vi "GetSubarrayOfCircularBuffer.vi"(8 "initialized array":waveform(dbl)[](array[waveform]), 9 "buffer size":i32, 10 "subset size":i32, 11 "start index":i32) -> (2 "initialized array 2":waveform(dbl)[](array[waveform]))   [LabVIEW 2016]
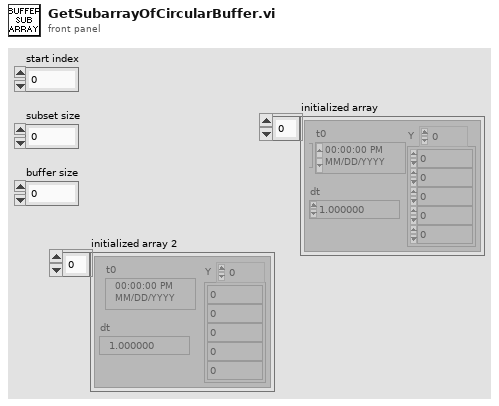
[diagram p1: front panel]
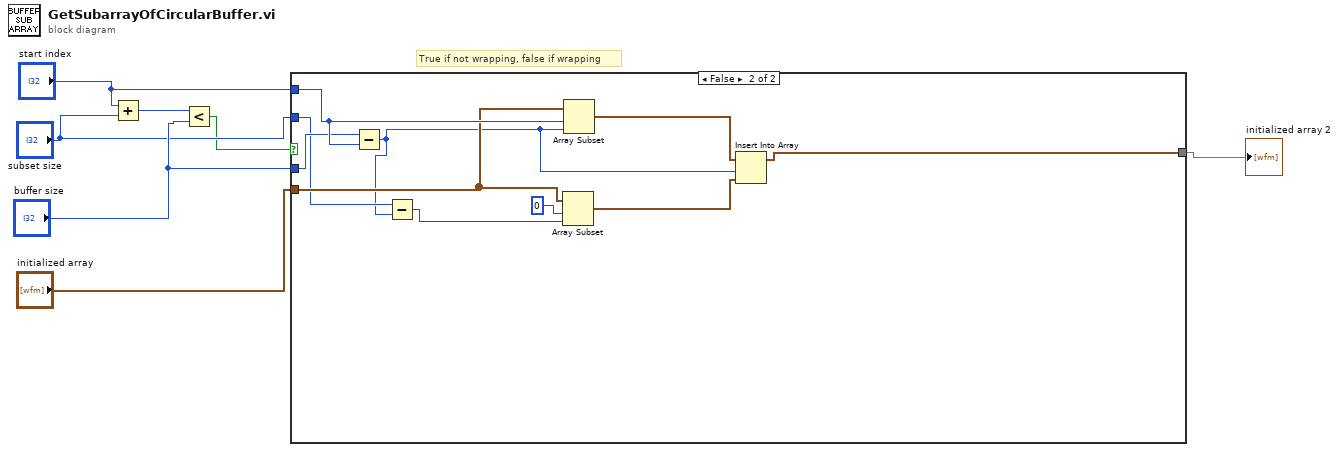
[diagram p0: block diagram]
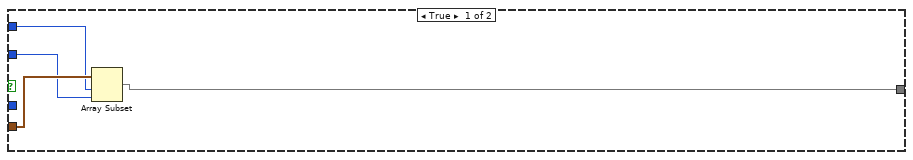
[diagram p2: hidden frame]
diagram:
  # "True if not wrapping, false if wrapping"
  n1 = Add(x="start index", y="subset size") -> (x+y=w3:i32)
  n2 = Less?(x=w3, y="buffer size") -> (x < y?=w4:bool)
  n3 = case shown="False" w4 {
    tunnel: "initialized array" -> [w11 w19]
    tunnel: "start index" -> [w10 w21]
    tunnel: "subset size" -> [w9 w17]
    tunnel: "buffer size" -> [_ w20]
    tunnel: [w8 w12] -> w1
    frame True {
      n4 = Array Subset(array=w11, index=w10, length=w9) -> (w8:waveform(dbl)[])
    }
    frame False, Default {
      n5 = Subtract(x=w20, y=w21) -> (x-y=w14:i32)
      n6 = Subtract(x=w17, y=w14) -> (x-y=w16:i32)
      n7 = Array Subset(array=w19, index=0, length=w16) -> (w13:waveform(dbl)[])
      n8 = Array Subset(array=w19, index=w21, length=w14) -> (w15:waveform(dbl)[])
      n9 = Insert Into Array(array=w15, index=w14, new element=w13) -> (w12:waveform(dbl)[])
    }
  }
  "initialized array 2" <- w1
